vi "Pixels number control.vi"(10 "samples acquired in":u32, 11 "Done?":bool) -> (3 "samples acquired out":u32)   [LabVIEW 2015]
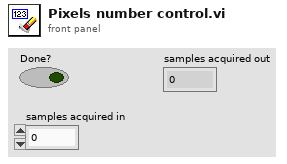
[diagram p1: front panel]
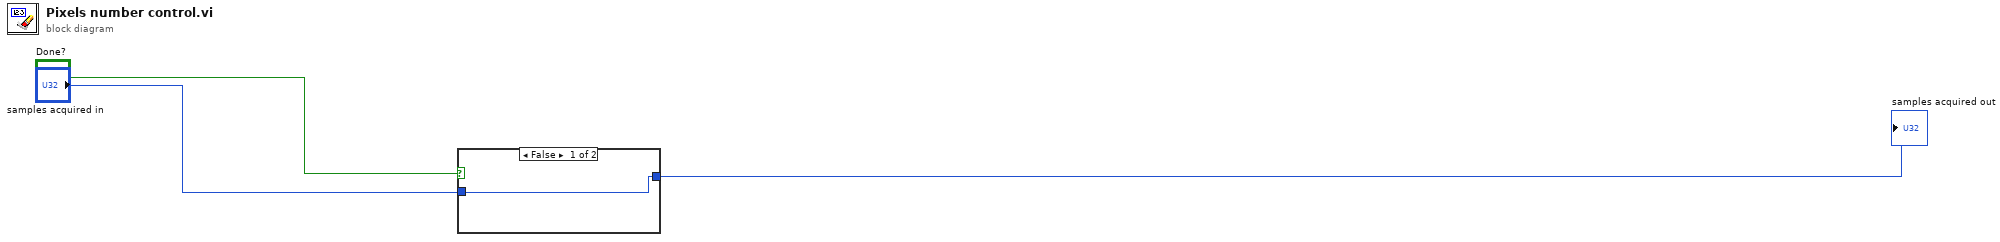
[diagram p0: block diagram]
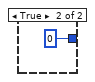
[diagram p2: hidden frame]
diagram:
  n1 = case shown="False" "Done?" {
    tunnel: "samples acquired in" -> [w4 _]
    tunnel: [w4 u32 0] -> w3
    frame False {
    }
    frame True {
    }
  }
  "samples acquired out" <- w3
